vi "Monitoring Real System.vi"() -> ()   [LabVIEW 2021]
panel:
  in  "File Path":path=path "C:/Temp/air_heater_data.lvm"
  in  "Record Button":bool
  out "Control Value [V]":dbl format="%.2g"
  out "Temperature [°C]":dbl format="%.1g"
  out "Control Chart":dbl(graph)=1.1724378087907898
  out "Measurement Chart":dbl(graph)
  in  "Stop":bool
  # "This Systems is Monitoring the Fuji PXG5 PID Controller Hardware Controlling the Real Air Heater System"
  # "Process Value (PV)"
  # "Manipulated Value (MV)"
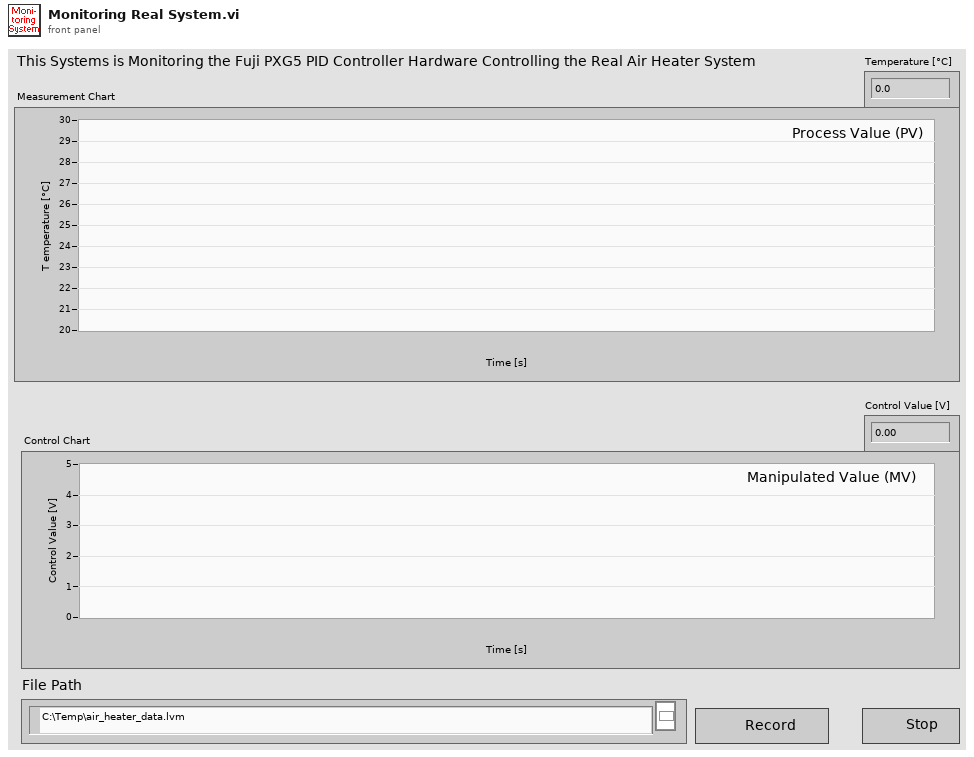
[diagram p1: front panel]
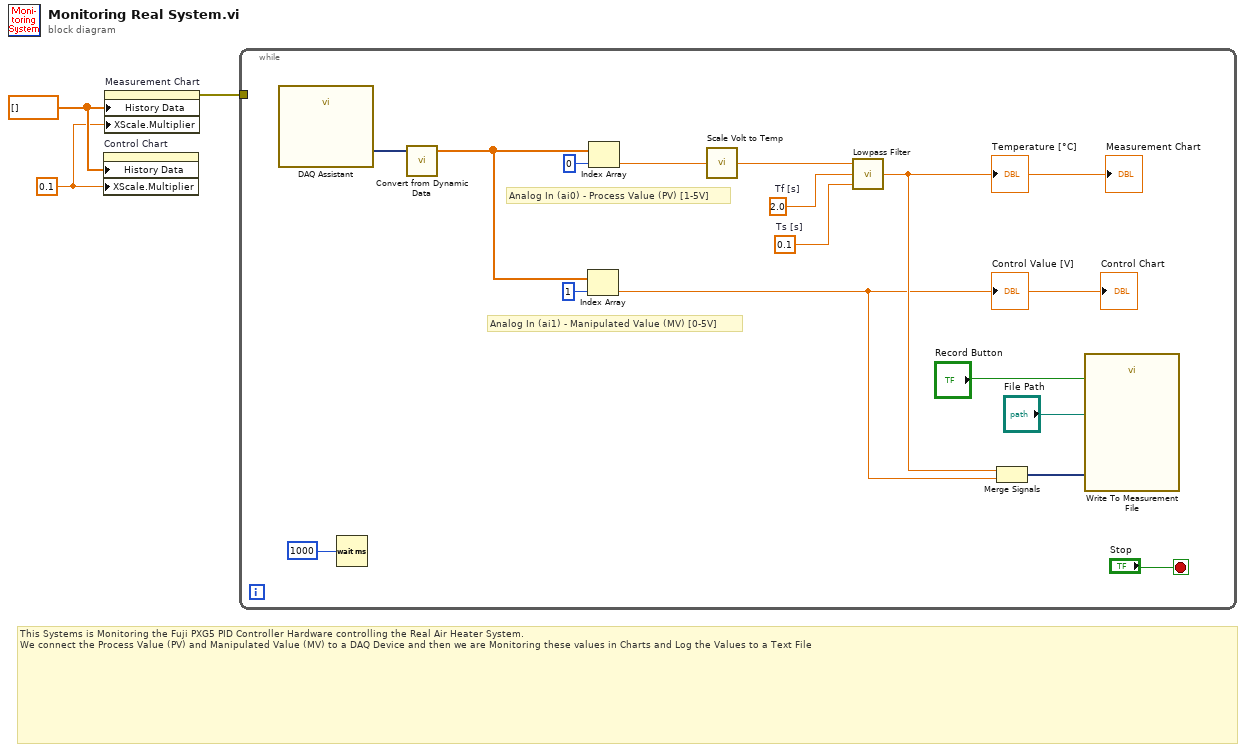
[diagram p0: block diagram]
diagram:
  w2 = 0.1 ("X Scale.Offset and Multiplier:Multiplier")
  w3 = dbl[] [] ("History Data")
  # "This Systems is Monitoring the Fuji PXG5 PID Controller Hardware controlling the Real Air Heater System.\nWe connect the Process Value (PV) and Manipulated Value (MV) to a DAQ Device and then we are Monitoring these values in Charts and Log the Values to a Text File"
  n1 = property on="Control Chart" class="WFChart (strict)"("History Data"=w3, "XScale.Multiplier"=w2) -> ()  [unwired: 2 in, 2 out]
  n2 = property on="Measurement Chart" class="WFChart (strict)"("History Data"=w3, "XScale.Multiplier"=w2) -> (error out=w1:errorcluster)  [unwired: 2 in, 1 out]
  n3 = while {
    tunnel: w1 -> [_]
    stop <- "Stop" stop-if-true
    w9 = 0.1  # Ts [s]
    w10 = 2.0  # Tf [s]
    # "Analog In (ai1) - Manipulated Value (MV) [0-5V]"
    # "Analog In (ai0) - Process Value (PV) [1-5V]"
    n4 = call "DAQ Assistant"() -> ("data"=w16:dynamicdata)  [unwired: 17 in, 2 out]
    n5 = Wait (ms)(milliseconds to wait=1000) -> ()  [unwired: 1 out]
    n6 = call "Convert from Dynamic Data"("Dynamic Data Type"=w16) -> ("Array"=w13:dbl[])  [unwired: 3 in]
    n7 = Index Array "Index Array"(array=w13, index=1) -> (element=w4:dbl)
    "Control Chart" <- w4
    "Control Value [V]" <- w4
    n8 = Index Array "Index Array"(array=w13, index=0) -> (element=w12:dbl)
    n9 = call "Scale Volt to Temp.vi"("Input Value [1-5V]"=w12) -> ("Output Value [20-50degC]"=w6:dbl)
    n10 = call "Lowpass Filter.vi"("Ts [s]"=w9, "Tf [s]"=w10, "Filter Input"=w6) -> ("Filter Output"=w5:dbl)
    "Measurement Chart" <- w5
    "Temperature [°C]" <- w5
    n11 = Merge Signals "Merge Signals"(w5, w4) -> (w11:dynamicdata)
    n12 = call "Write To Measurement File"("Signals"=w11, "Enable"="Record Button", "Filename"="File Path") -> ()  [unwired: 14 in, 3 out]
  }
